vi "digital read.vi"(8 "error in (no error)":errorcluster, 10 "Line":string, 11 "USB IO in":refnum<class "USB IO.lvclass">) -> (0 "error out":errorcluster, 2 "High/Low":bool, 3 "USB IO out":refnum<class "USB IO.lvclass">)   [LabVIEW 2025, in "USB IO.lvlib" / "USB IO.lvclass"]
uses:
  USB IO.lvclass
  USB IO.lvclass/USB IO.ctl
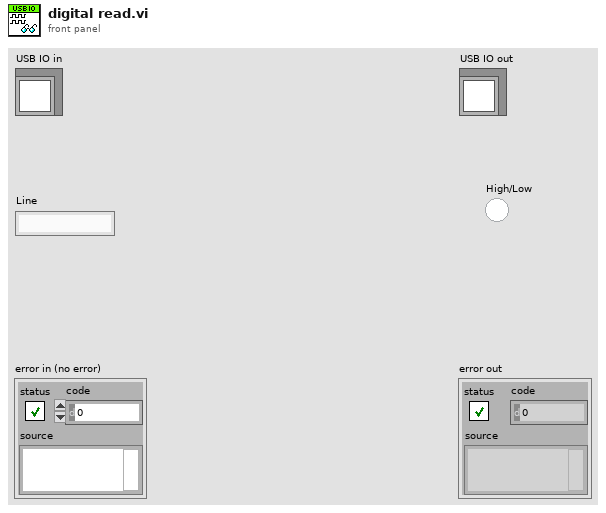
[diagram p1: front panel]
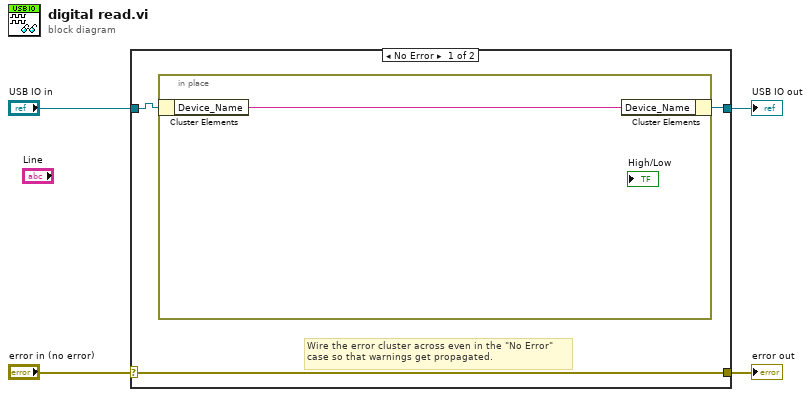
[diagram p0: block diagram]
diagram:
  n1 = case shown="No Error" "error in (no error)" {
    selector: "error in (no error)" -> [w7 w10]
    tunnel: [w7 w10] -> w3
    tunnel: [w5 w9] -> w1
    tunnel: "USB IO in" -> [w6 w9]
    frame No Error {
      # "Wire the error cluster across even in the \"No Error\"\ncase so that warnings get propagated."
      n2 = in-place {
        n3 = in-place-cluster #1(w6) -> ("Device_Name"=w8:string)
        n4 = in-place-cluster #1("Device_Name"=w8) -> (w5:refnum<class "USB IO.lvclass">)
      }
    }
    frame Error {
    }
  }
  "error out" <- w3
  "USB IO out" <- w1
